vi "Wago Update Voltage Adjustment Parameters.vi"(8 "error in (no error)":errorcluster, 10 "Voltage Adjustment Parameters":T1, 11 "Modbus Master in":refnum<class "Modbus Master.lvclass">) -> (0 "error out":errorcluster, 3 "Modbus master out":refnum<class "Modbus Master.lvclass">)   [LabVIEW 2016]
uses:
  Type Definitions/Wago Voltage Adjustment Parameters.ctl
  <vilib>/NI/Modbus Library/API/Master/Modbus Master.lvclass
panel:
  out "Voltage Adjustment Parameters":T1
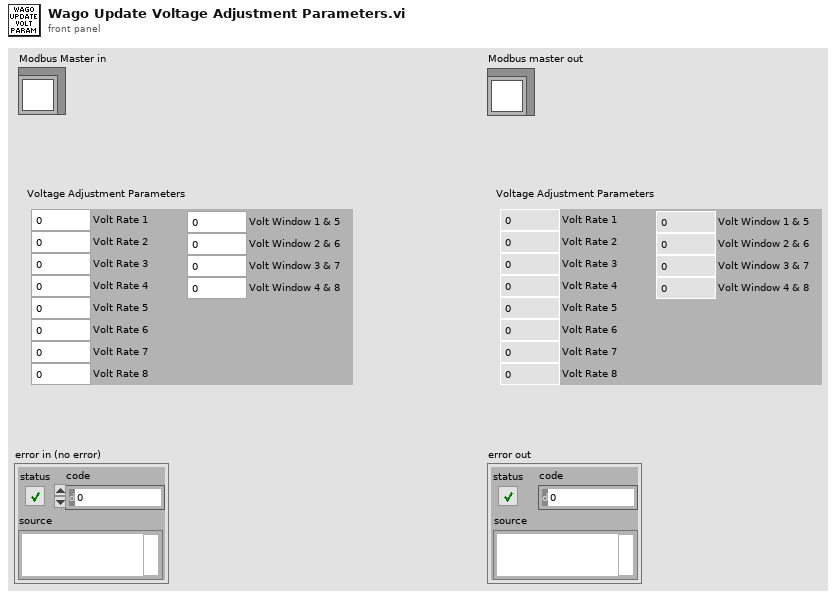
[diagram p1: front panel]
types:
  T1 = typedef "Wago Voltage Adjustment Parameters.ctl" = cluster{"Volt Rate 1":u16, "Volt Rate 2":u16, "Volt Rate 3":u16, "Volt Rate 4":u16, "Volt Rate 5":u16, "Volt Rate 6":u16, "Volt Rate 7":u16, "Volt Rate 8":u16, "Volt Window 1 & 5":u16, "Volt Window 2 & 6":u16, "Volt Window 3 & 7 ":u16, "Volt Window 4 & 8":u16}
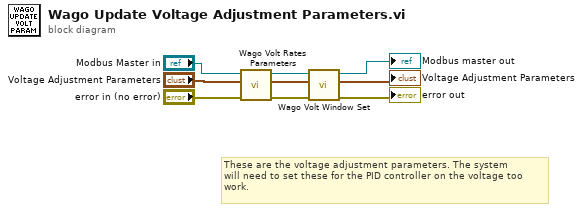
[diagram p0: block diagram]
diagram:
  # "These are the voltage adjustment parameters. The system \nwill need to set these for the PID controller on the voltage too\nwork."
  n1 = call "Wago Volt Rates Parameters.vi"("error in (no error)"="error in (no error)", "Voltage Adjustment Parameters"="Voltage Adjustment Parameters", "Modbus Master in"="Modbus Master in") -> ("error out"=w4:errorcluster, "Modbus Master out"=w5:refnum<class "Modbus Master.lvclass">)  [unwired: 7 in]
  n2 = call "Wago Volt Window Set.vi"("error in (no error)"=w4, "Voltage Adjustment Parameters in"="Voltage Adjustment Parameters", "Modbus Master in"=w5) -> ("error out"=→"error out":errorcluster, "Voltage Adjustment Parameters out"=→"Voltage Adjustment Parameters":T1, "Modbus Master out"=→"Modbus master out":refnum<class "Modbus Master.lvclass">)  [unwired: 6 in]
